vi "main.vi"(0 "Operations":string(tree), 1 "Add":bool, 3 "Delete":bool, 11 "Error In":errorcluster, 12 "Save Data":bool, 13 "Load Data":bool, 14 "Operation List":string(combo)="Add") -> (15 "Error Out":errorcluster)   [LabVIEW 2020, in "Calculator_Using_Objects.lvlib"]
doc: "This VI is to perform the math operations. Whereas the history of the operations will be saved in objects. \nThey can be retrived from the memory during the start of the VI."
uses:
  Calculator_Using_Objects.lvlib
  Typedef's/Q_Operations.ctl
  Typedef's/Data_Cluster.ctl
  Classes/Arithmetic_Operations/Arithmetic_Operations.lvclass
  Typedef's/UserEvent_Operations.ctl
  Classes/Children/Add/Add.lvclass
  Classes/Children/Divide/Divide.lvclass
  Classes/Children/Multiplication/Multiplication.lvclass
  Classes/Children/Subtract/Subtract.lvclass
  Typedef's/Event_Data.ctl
  Typedef's/Object_And_Name_Cluster.ctl
  <vilib>/Utility/error.llb/DialogType.ctl
  <vilib>/Utility/xml.llb/Write to XML File(string).vi
  <vilib>/Utility/xml.llb/Read From XML File(string).vi
panel:
  # "Description:\n1. The classes that were present in the children folder in classes will be automatically loaded into the Operation List box. \n2. Double click any one of it and press add button to add once instance of that particular operation into the Operations box. \n3. Once the operation is clicked the particular instance operation method will be loaded into the subpanel. Where it will have the controls to perform \nthe operations.\n4. The delete button will delete that particular instance of operation in the Operations. \n5. The Save Data button will save all the data instances into a file which can be loaded later. \n6. The Load button will load the data that is already stored in the disc. Loading data will clear all the existing data."
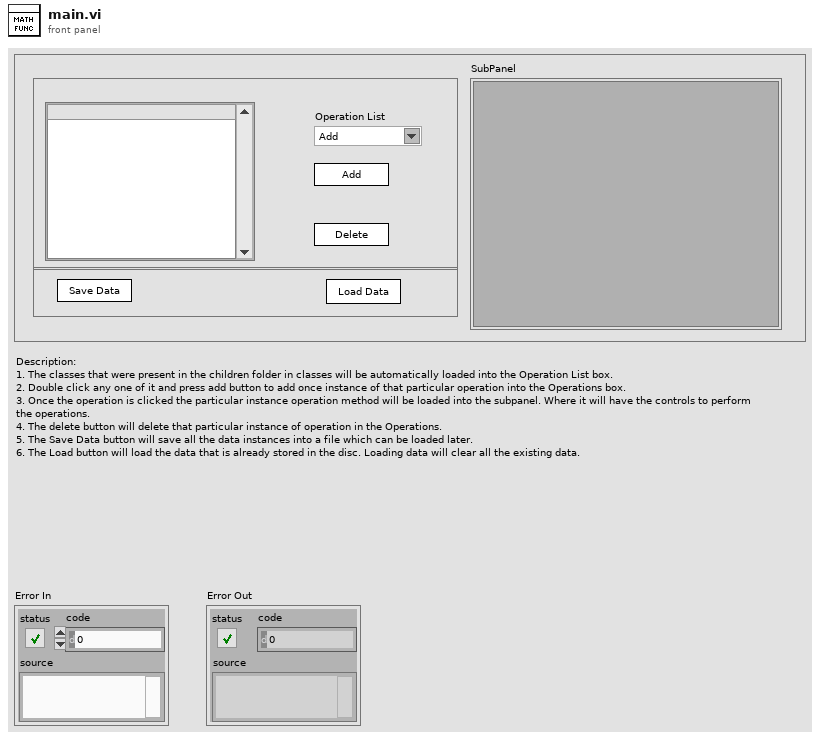
[diagram p1: front panel]
types:
  T1 = typedef "Calculator_Using_Objects.lvlib/UserEvent_Operations.ctl" = enum16{"Create", "Generate", "Get Ref", "Destroy"}
  T2 = typedef "Calculator_Using_Objects.lvlib/Data_Cluster.ctl" = cluster{"Operation Selected":string, "Objects Array":refnum<class "Arithmetic_Operations.lvclass">[], "Prev Row Number":i32, "Num 1":dbl, "Num 2":dbl, "Application Path":path, "Row Number":i32, "Subpanel FP?":bool}
  T3 = typedef "Calculator_Using_Objects.lvlib/Q_Operations.ctl" = enum16{"Create Q", "Enqueue", "Dequeue", "Enqueue N ele", "Enstack N ele", "Flush Q", "Destroy Q"}
  T4 = typedef "Calculator_Using_Objects.lvlib/Event_Data.ctl" = cluster{"Stop Data":bool}
  T5 = typedef "Calculator_Using_Objects.lvlib/Object_And_Name_Cluster.ctl" = cluster{"Tree Entry":string[], "Object Array":refnum<class "Arithmetic_Operations.lvclass">[]}
  T6 = enum16{"open", "replace", "create", "open or create", "replace or create", "replace or create with confirmation"}
  T7 = typedef "DialogType.ctl" = u16
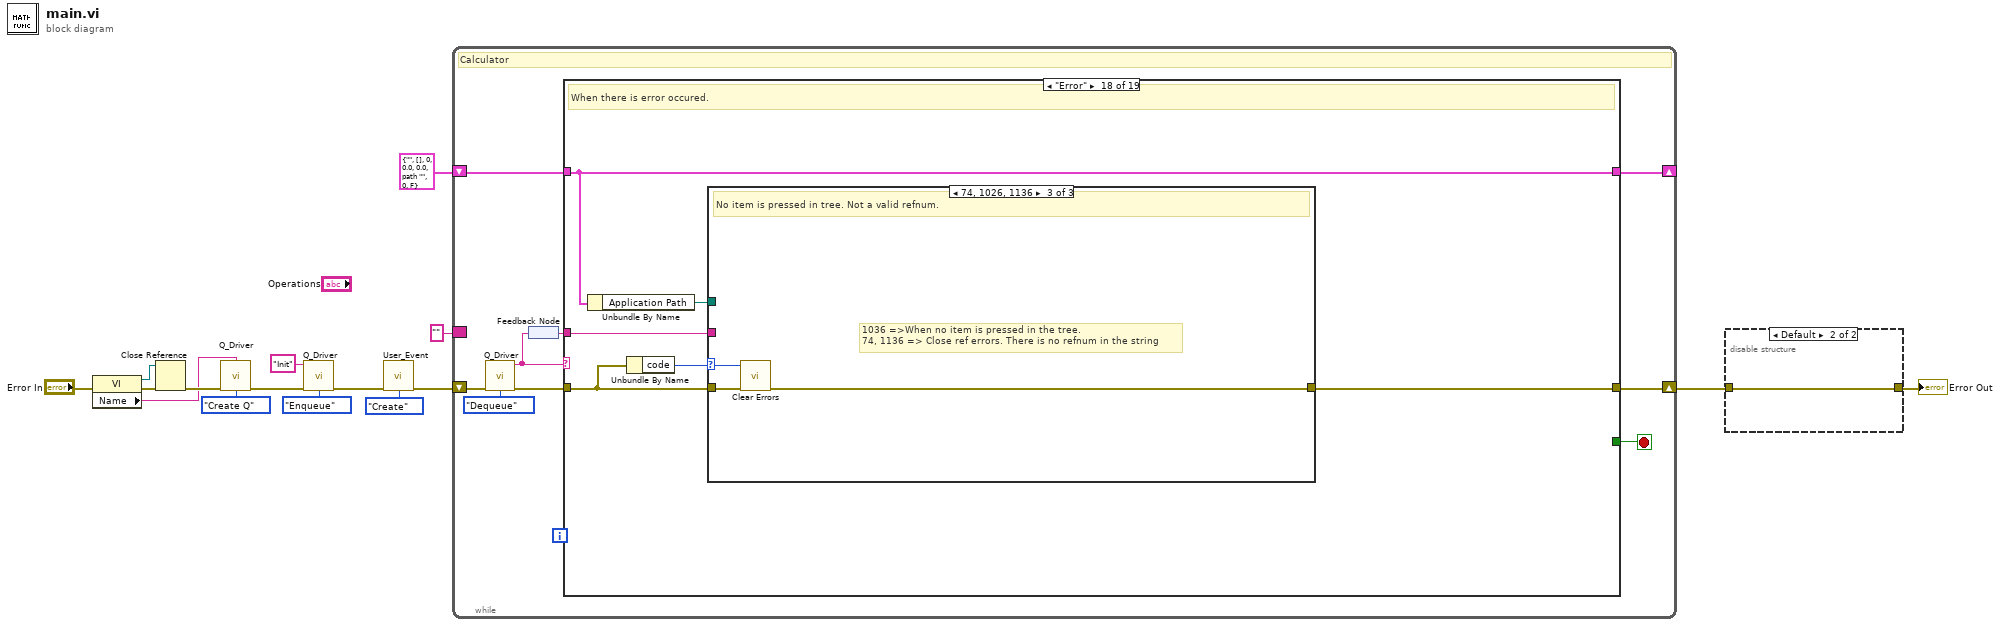
[diagram p0: block diagram]
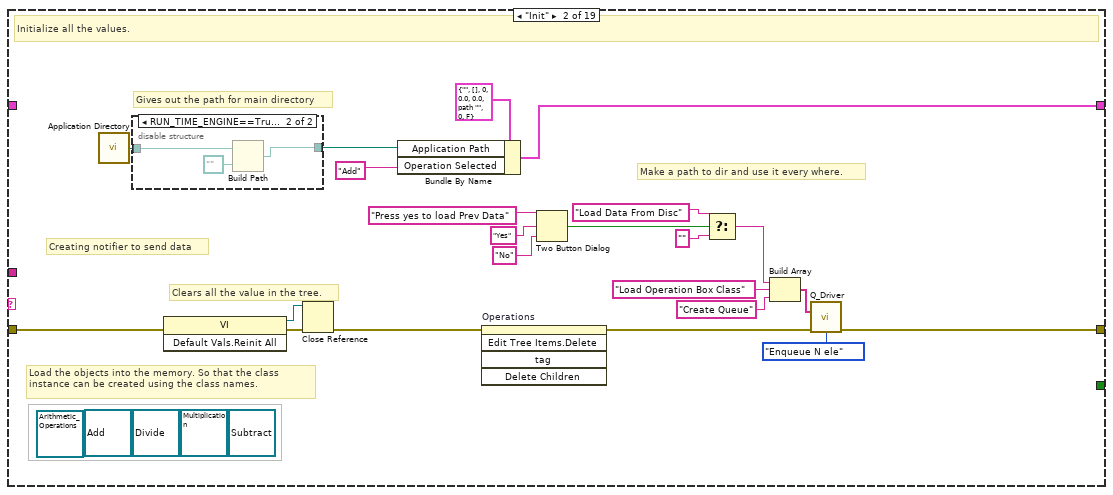
[diagram p3: hidden frame]
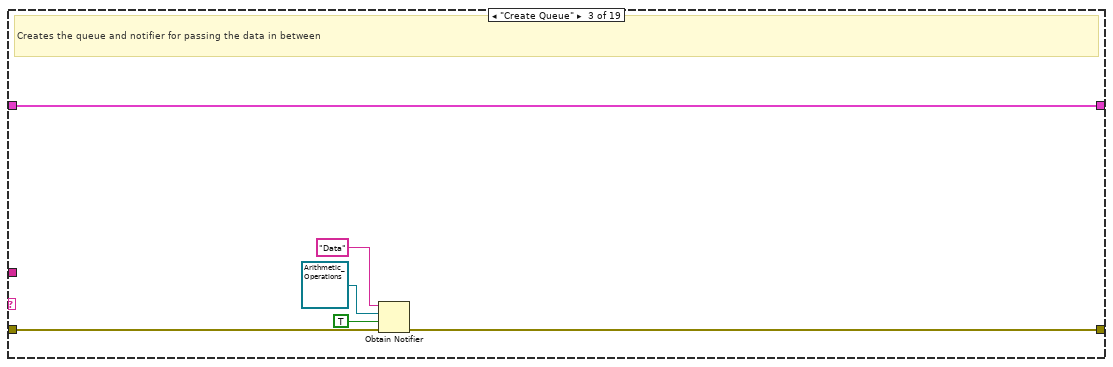
[diagram p5: hidden frame]
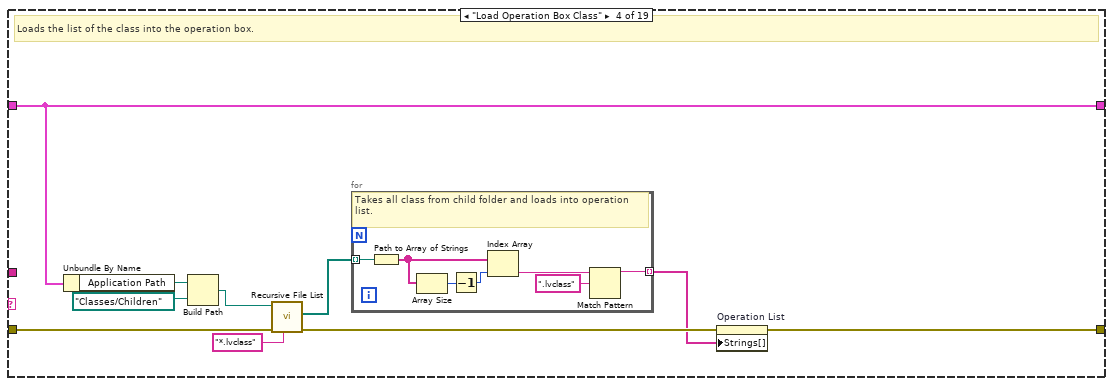
[diagram p6: hidden frame]
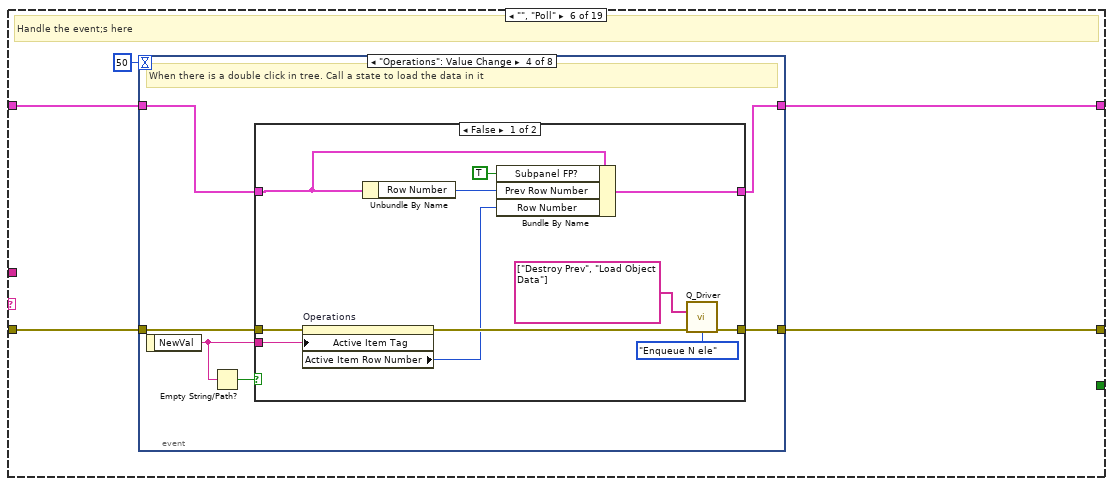
[diagram p8: hidden frame]
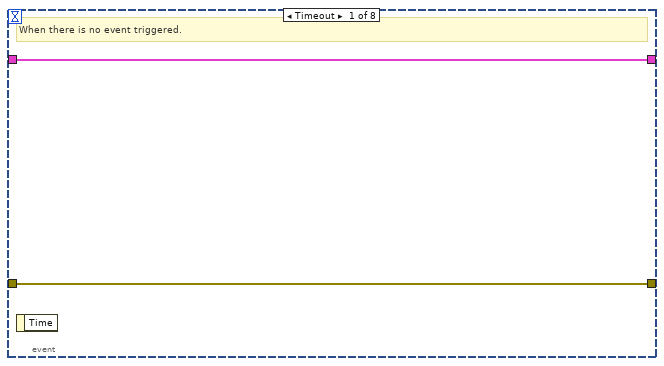
[diagram p9: hidden frame]
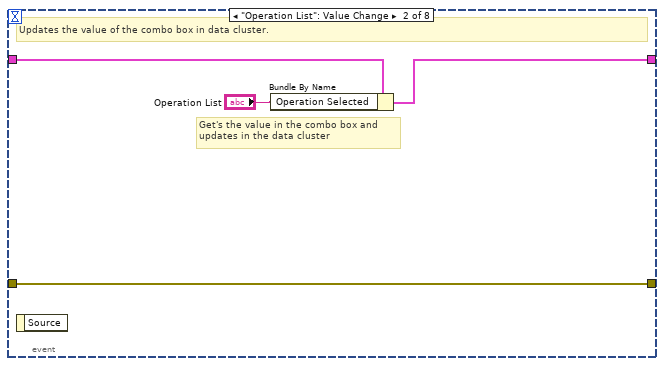
[diagram p10: hidden frame]
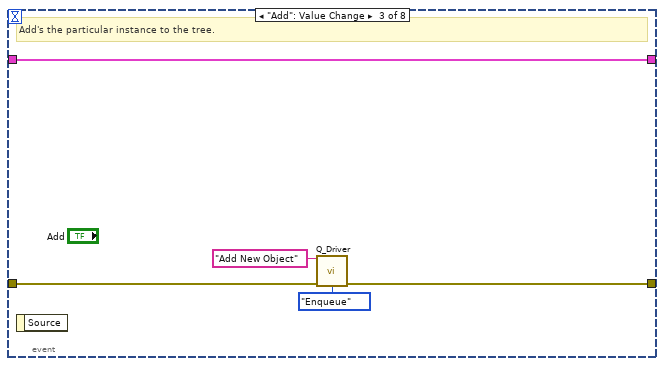
[diagram p11: hidden frame]
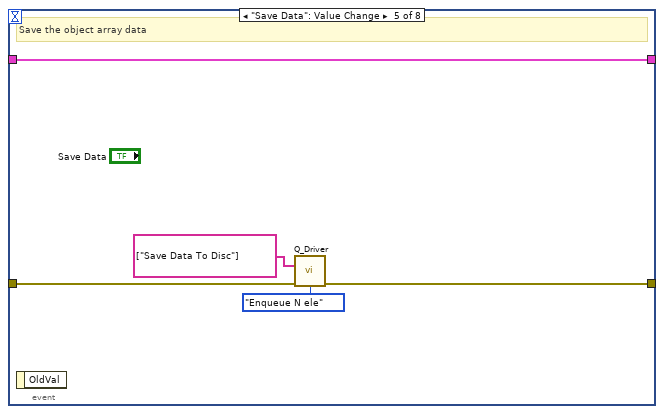
[diagram p13: hidden frame]
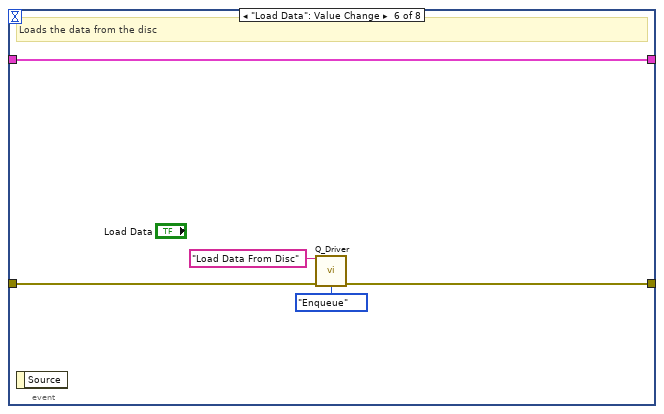
[diagram p14: hidden frame]
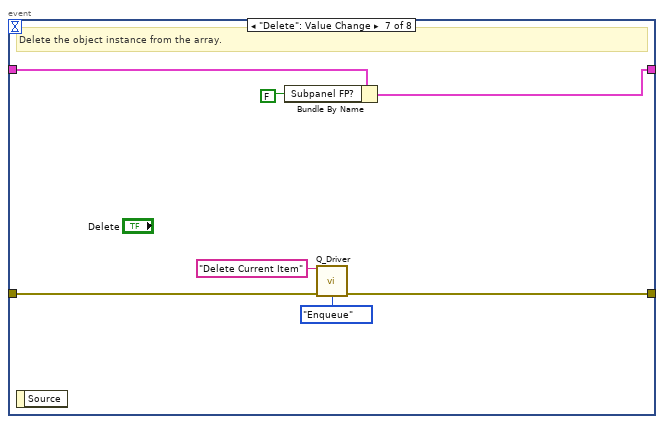
[diagram p15: hidden frame]
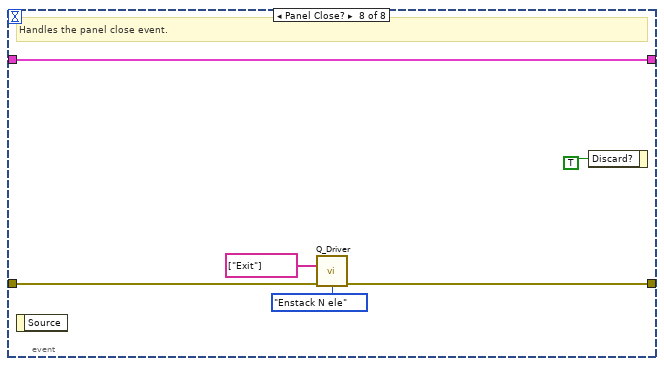
[diagram p16: hidden frame]
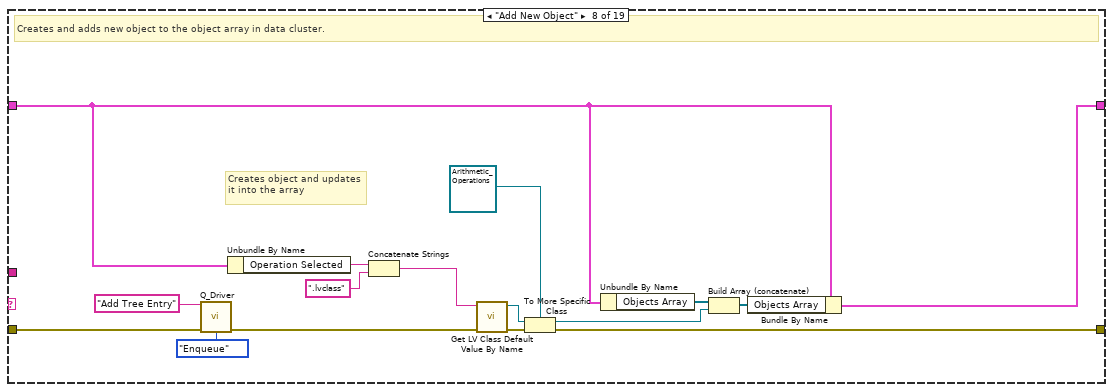
[diagram p18: hidden frame]
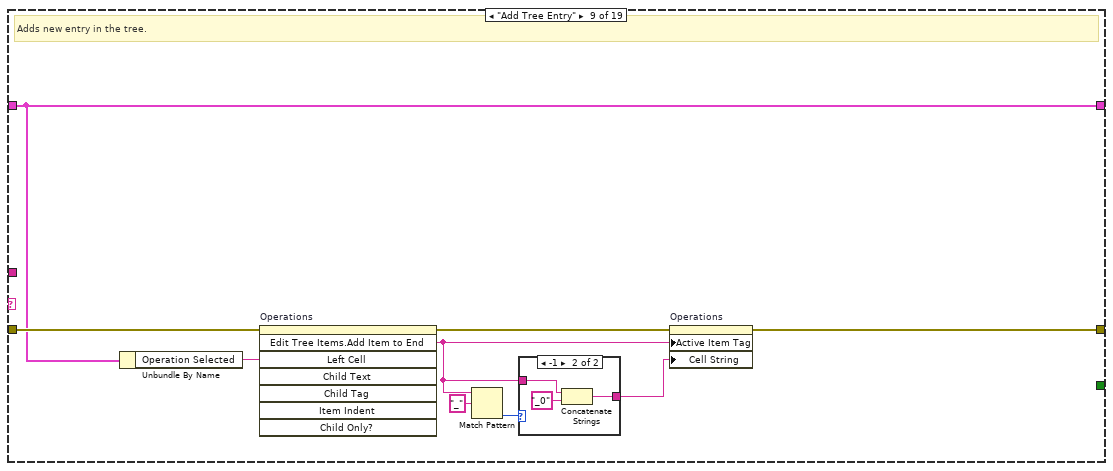
[diagram p19: hidden frame]
diagram:
  n1 = property class="VI"(error in="Error In") -> (reference out=w13:refnum<vi>, error out=w15:errorcluster, "Name"=w10:string)  [unwired: 1 in]
  n2 = Close Reference(reference=w13, error in (no error)=w15) -> (error out=w14:errorcluster)
  n3 = call "Q_Driver.vi"("Name"=w10, "Error In"=w14, "Operations"=Q_Operations."Create Q") -> ("Error Out"=w12:errorcluster)  [unwired: 11 in, 1 out]
  n4 = call "Q_Driver.vi"("State"="Init", "Error In"=w12, "Operations"=Q_Operations."Enqueue") -> ("Error Out"=w9:errorcluster)  [unwired: 11 in, 1 out]
  n5 = call "User_Event.vi"("Error In"=w9, "Enum"=UserEvent_Operations."Create") -> ("Error Out"=w6:errorcluster)  [unwired: 12 in, 1 out]
  n6 = while {
    shift-right: [w22] -> w4
    shift-left: w6 -> [w24]
    shift-right: [w19] -> _
    shift-left: T2 {"Operation Selected"="", "Objects Array"=[], "Prev Row Number"=0, "Num 1"=0.0, "Num 2"=0.0, "Application Path"=path "", "Row Number"=0, "Subpanel FP?"=FALSE} ("Data Cluster") -> [w20]
    border: "" ("Dequeued Element") -> [_]
    stop <- w21 stop-if-true
    # "Calculator"
    n7 = call "Q_Driver.vi"("Error In"=w24, "Operations"=Q_Operations."Dequeue") -> ("Dequeued Element"=w18:string, "Error Out"=w25:errorcluster)  [unwired: 12 in]
    n8 = feedback-in #1(w18) -> ()
    n9 = feedback #1() -> (w17:string)
    n10 = case shown="\"Error\"" w18 {
      tunnel: w25 -> [w27 w37 w54 w69 w78 w82 w138 w154 w163 w172 w198 w201 w211 w251 w259 w267 w281 w286 w330]
      tunnel: [w27 w42 w55 w65 w78 w81 w138 w153 w157 w171 w196 w206 w212 w244 w259 w264 w281 w287 w330] -> w22
      tunnel: [_ _ _ _ _ _ _ _ _ _ _ _ _ _ _ TRUE _ _ _] -> w21
      tunnel: w20 -> [w26 _ w59 w63 w77 w80 w137 w151 w161 w168 w197 w207 w209 w249 w258 w261 w280 w284 w329]
      tunnel: [w26 w33 w59 w63 w77 w79 w137 w148 w161 w169 w195 w207 w210 w245 w258 w261 w280 w284 w329] -> w19
      tunnel: w17 -> [_ _ _ _ _ _ _ _ _ _ _ _ _ _ _ _ _ w282 _]
      frame "/**** Initialize ****/" {
      }
      frame "Init" {
        (unwired) refnum<class "Subtract.lvclass"> refnum ("Subtract.lvclass")
        (unwired) refnum<class "Multiplication.lvclass"> refnum ("Multiplication.lvclass")
        (unwired) refnum<class "Divide.lvclass"> refnum ("Divide.lvclass")
        (unwired) refnum<class "Add.lvclass"> refnum ("Add.lvclass")
        (unwired) refnum<class "Arithmetic_Operations.lvclass"> refnum ("Arithmetic_Operations.lvclass")
        # "Creating notifier to send data"
        # "Load the objects into the memory. So that the class instance can be created using the class names."
        # "Gives out the path for main directory"
        # "Make a path to dir and use it every where."
        # "Clears all the value in the tree."
        # "Initialize all the values."
        n11 = call <vilib>:"Application Directory.vi"() -> ("Application Directory"=w31:path)
        n12 = disable-structure shown="RUN_TIME_ENGINE==True" {
          disable-tunnel: [w50 w51] -> w32
          disable-tunnel: w31 -> [w50 w53]
          frame condition #0 (active) {
          }
          frame condition #1 {
            n13 = Build Path(base path=w53, name or relative path=path "..") -> (appended path=w51:path)
          }
        }
        n14 = invoke class="VI" method="Default Vals.Reinit All"(error in=w37) -> (reference out=w48:refnum<vi>, error out=w49:errorcluster)  [unwired: 2 in, 1 out]
        n15 = Close Reference(reference=w48, error in (no error)=w49) -> (error out=w47:errorcluster)
        n16 = Bundle By Name(cluster=T2 {"Operation Selected"="", "Objects Array"=[], "Prev Row Number"=0, "Num 1"=0.0, "Num 2"=0.0, "Application Path"=path "", "Row Number"=0, "Subpanel FP?"=FALSE} ("Data Cluster"), "Application Path"=w32, "Operation Selected"="Add") -> (w33:T2)
        n17 = invoke on="Operations" class="Tree (strict)" method="Edit Tree Items.Delete"(error in=w47) -> (error out=w43:errorcluster)  [unwired: 4 in, 4 out]
        n18 = Two Button Dialog(message="Press yes to load Prev Data", 1:"No" ("F button name (\"Cancel\")"), 2:"Yes" ("T button name (\"OK\")")) -> (T button?=w41:bool)
        n19 = Select(t="Load Data From Disc", s=w41, f="") -> (s? t:f=w36:string)
        n20 = Build Array(w36, "Load Operation Box Class", "Create Queue") -> (w34:string[])
        n21 = call "Q_Driver.vi"("States[]"=w34, "Error In"=w43, "Operations"=Q_Operations."Enqueue N ele") -> ("Error Out"=w42:errorcluster)  [unwired: 11 in, 1 out]
      }
      frame "Create Queue" {
        # "Creates the queue and notifier for passing the data in between"
        n22 = Obtain Notifier(name (unnamed)="Data", notification data type=refnum<class "Arithmetic_Operations.lvclass"> refnum ("Arithmetic_Operations.lvclass"), create if not found? (T)=TRUE, error in (no error)=w54) -> (error out=w55:errorcluster)  [unwired: 2 out]
      }
      frame "Load Operation Box Class" {
        # "Loads the list of the class into the operation box."
        n23 = Unbundle By Name(w63) -> ("Application Path"=w61:path)
        n24 = Build Path(base path=w61, name or relative path=path "Classes/Children") -> (appended path=w60:path)
        n25 = call <vilib>:"Recursive File List.vi"("pattern"="*.lvclass", "error in (no error)"=w69, "Folder Path"=w60) -> ("error out"=w68:errorcluster, "All Files in Dir"=w66:path[])  [unwired: 4 in, 3 out]
        n26 = for {
          tunnel: w66 -> [w76] mode=indexing
          tunnel: [w70] -> w64 mode=indexing
          # "Takes all class from child folder and loads into operation list."
          n27 = Path to Array of Strings(0:w76) -> (2:w74:string[])  [unwired: 1 out]
          n28 = Array Size(array=w74) -> (size(s)=w75:i32)
          n29 = Decrement(x=w75) -> (x-1=w73:i32)
          n30 = Index Array(array=w74, index=w73) -> (element=w72:string)
          n31 = Match Pattern(string=w72, regular expression=".lvclass") -> (before substring=w70:string)  [unwired: 1 in, 3 out]
        }
        n32 = property on="Operation List" class="CmbBox"(error in=w68, "Strings[]"=w64) -> (error out=w65:errorcluster)  [unwired: 1 in, 1 out]
      }
      frame "/****Events*****/" {
      }
      frame "", "Poll" {
        # "Handle the event;s here"
        n33 = event shown="[3] \"Operations\": Value Change" {
          selector: _ -> [_ _ _ _ _ _ _ _]
          dyn-events: _ -> [_ _ _ _ _ _ _ _]
          timeout: 50 -> [_ _ _ _ _ _ _ _]
          tunnel: w82 -> [w85 w89 w94 w99 w118 w123 w130 w136]
          tunnel: [w85 w89 w92 w100 w116 w121 w128 w134] -> w81
          tunnel: [w84 w87 w93 w96 w117 w122 w125 w131] -> w79
          tunnel: w80 -> [w84 w88 w93 w97 w117 w122 w129 w131]
          event Timeout {
            # "When there is no event triggered."
            n34 = event-data() -> ()  [unwired: 1 in, 1 out]
          }
          event "Operation List": Value Change {
            # "Get's the value in the combo box and\nupdates in the data cluster"
            # "Updates the value of the combo box in data cluster."
            n35 = event-data() -> ()  [unwired: 1 in, 1 out]
            n36 = Bundle By Name(cluster=w88, "Operation Selected"="Operation List") -> (w87:T2)
          }
          event "Add": Value Change {
            # "Add's the particular instance to the tree."
            n37 = event-data() -> ()  [unwired: 1 in, 1 out]
            n38 = call "Q_Driver.vi"("State"="Add New Object", "Error In"=w94, "Operations"=Q_Operations."Enqueue") -> ("Error Out"=w92:errorcluster)  [unwired: 11 in, 1 out]
          }
          event "Operations": Value Change {
            # "When there is a double click in tree. Call a state to load the data in it"
            n39 = event-data() -> ("NewVal"=w98:string)  [unwired: 1 in]
            n40 = Empty String/Path?(string/path=w98) -> (empty?=w95:bool)
            n41 = case shown="False" w95 {
              tunnel: [w111 w113] -> w100
              tunnel: [w110 w112] -> w96
              tunnel: w99 -> [w106 w113]
              tunnel: w98 -> [w104 _]
              tunnel: w97 -> [w101 w112]
              frame False {
                n42 = property on="Operations" class="Tree (strict)"(error in=w106, "Active Item Tag"=w104) -> (error out=w109:errorcluster, "Active Item Row Number"=w108:i32)  [unwired: 1 in, 1 out]
                n43 = Unbundle By Name(w101) -> ("Row Number"=w107:i32)
                n44 = Bundle By Name(cluster=w101, "Subpanel FP?"=TRUE, "Prev Row Number"=w107, "Row Number"=w108) -> (w110:T2)
                n45 = call "Q_Driver.vi"("States[]"=string[] ["Destroy Prev", "Load Object Data"], "Error In"=w109, "Operations"=Q_Operations."Enqueue N ele") -> ("Error Out"=w111:errorcluster)  [unwired: 11 in, 1 out]
              }
              frame True {
              }
            }
          }
          event "Save Data": Value Change {
            # "Save the object array data"
            n46 = event-data() -> ()  [unwired: 1 in, 1 out]
            n47 = call "Q_Driver.vi"("States[]"=string[] ["Save Data To Disc"], "Error In"=w118, "Operations"=Q_Operations."Enqueue N ele") -> ("Error Out"=w116:errorcluster)  [unwired: 11 in, 1 out]
          }
          event "Load Data": Value Change {
            # "Loads the data from the disc"
            n48 = event-data() -> ()  [unwired: 1 in, 1 out]
            n49 = call "Q_Driver.vi"("State"="Load Data From Disc", "Error In"=w123, "Operations"=Q_Operations."Enqueue") -> ("Error Out"=w121:errorcluster)  [unwired: 11 in, 1 out]
          }
          event "Delete": Value Change {
            # "Delete the object instance from the array."
            n50 = event-data() -> ()  [unwired: 1 in, 1 out]
            n51 = Bundle By Name(cluster=w129, "Subpanel FP?"=FALSE) -> (w125:T2)
            n52 = call "Q_Driver.vi"("State"="Delete Current Item", "Error In"=w130, "Operations"=Q_Operations."Enqueue") -> ("Error Out"=w128:errorcluster)  [unwired: 11 in, 1 out]
          }
          event Panel Close? {
            # "Handles the panel close event."
            n53 = event-data() -> ()  [unwired: 1 in, 1 out]
            n54 = call "Q_Driver.vi"("States[]"=string[] ["Exit"], "Error In"=w136, "Operations"=Q_Operations."Enstack N ele") -> ("Error Out"=w134:errorcluster)  [unwired: 11 in, 1 out]
            n55 = event-data("Discard?"=TRUE) -> ()  [unwired: 1 in, 1 out]
          }
        }
      }
      frame "/**** Functionalities ***/" {
      }
      frame "Add New Object" {
        # "Creates object and updates it into the array"
        # "Creates and adds new object to the object array in data cluster."
        n56 = call "Q_Driver.vi"("State"="Add Tree Entry", "Error In"=w154, "Operations"=Q_Operations."Enqueue") -> ("Error Out"=w146:errorcluster)  [unwired: 11 in, 1 out]
        n57 = Unbundle By Name(w151) -> ("Operation Selected"=w141:string)
        n58 = Concatenate Strings(w141, ".lvclass") -> (w139:string)
        n59 = call <vilib>:"Get LV Class Default Value By Name.vi"("error in (no error)"=w146, "class name"=w139) -> ("error out"=w143:errorcluster, "object"=w142:refnum<class>)  [unwired: 8 in]
        n60 = To More Specific Class(target class=refnum<class "Arithmetic_Operations.lvclass"> refnum ("Arithmetic_Operations.lvclass"), reference=w142, error in=w143) -> (specific class reference=w149:refnum<class "Arithmetic_Operations.lvclass">, error out=w153:errorcluster)
        n61 = Unbundle By Name(w151) -> ("Objects Array"=w150:refnum<class "Arithmetic_Operations.lvclass">[])
        n62 = Build Array (concatenate)(w150, w149) -> (w147:refnum<class "Arithmetic_Operations.lvclass">[])
        n63 = Bundle By Name(cluster=w151, "Objects Array"=w147) -> (w148:T2)
      }
      frame "Add Tree Entry" {
        # "Adds new entry in the tree."
        n64 = Unbundle By Name(w161) -> ("Operation Selected"=w162:string)
        n65 = invoke on="Operations" class="Tree (strict)" method="Edit Tree Items.Add Item to End"(error in=w163, "Left Cell"=w162) -> (error out=w158:errorcluster, "Edit Tree Items:Add Item to End"=w156:string)  [unwired: 6 in, 6 out]
        n66 = Match Pattern(string=w156, regular expression="_") -> (offset past match=w159:i32)  [unwired: 1 in, 3 out]
        n67 = case shown="-1" w159 {
          tunnel: w156 -> [w164 w166]
          tunnel: [w164 w165] -> w155
          frame 0, Default {
          }
          frame -1 {
            n68 = Concatenate Strings(w166, "_0" ("string")) -> (w165:string)
          }
        }
        n69 = property on="Operations" class="Tree (strict)"(error in=w158, "Active Item Tag"=w156, "Cell String"=w155) -> (error out=w157:errorcluster)  [unwired: 1 in, 1 out]
      }
      frame "Destroy Prev" {
        # "Destroy's the prev operation using the event."
        n70 = First Call?() -> (First Call?: T/F=w170:bool)
        n71 = case shown="False" w170 {
          tunnel: w172 -> [w185 w187]
          tunnel: [w173 w187] -> w171
          tunnel: w168 -> [w181 w186]
          tunnel: [w175 w186] -> w169
          frame False {
            # "After first call do these operation."
            n72 = invoke on="SubPanel" class="SubPnl" method="Remove VI"(error in=w185) -> (error out=w184:errorcluster)  [unwired: 2 in, 2 out]
            n73 = Unbundle By Name(w181) -> ("Objects Array"=w178:refnum<class "Arithmetic_Operations.lvclass">[], "Prev Row Number"=w176:i32)
            n74 = call "User_Event.vi"("Event Data"=T4 {"Stop Data"=TRUE}, "Error In"=w184, "Enum"=UserEvent_Operations."Generate") -> ("Error Out"=w179:errorcluster)  [unwired: 11 in, 1 out]
            n75 = Index Array(array=w178, index=w176) -> (element=w180:refnum<class "Arithmetic_Operations.lvclass">)
            n76 = call-dynamic "Get_Data.vi"("Arithmetic_Operations in"=w180, "Error In"=w179) -> ("Arithmetic_Operations out"=w177:refnum<class "Arithmetic_Operations.lvclass">, "Error Out"=w173:errorcluster)  [unwired: 12 in]
            n77 = Replace Array Subset(array=w178, new element=w177, index=w176) -> (w174:refnum<class "Arithmetic_Operations.lvclass">[])
            n78 = Bundle By Name(cluster=w181, "Objects Array"=w174) -> (w175:T2)
          }
          frame True {
            # "During first call do nothing."
          }
        }
      }
      frame "Load Object Data" {
        # "Loads the object data into the front panel."
        n79 = property on="Operations" class="Tree (strict)"(error in=w198) -> (error out=w188:errorcluster, "Active Item Row Number"=w193:i32)  [unwired: 1 in, 1 out]
        n80 = Unbundle By Name(w197) -> ("Objects Array"=w194:refnum<class "Arithmetic_Operations.lvclass">[])
        n81 = Index Array(array=w194, index=w193) -> (element=w190:refnum<class "Arithmetic_Operations.lvclass">)
        n82 = control-ref of="SubPanel"() -> (w189:refnum<vi>)
        n83 = call-dynamic "Talker.vi"("Arithmetic_Operations in"=w190, "Subpanel Ref"=w189, "Error In"=w188) -> ("Arithmetic_Operations out"=w191:refnum<class "Arithmetic_Operations.lvclass">, "Error Out"=w196:errorcluster)  [unwired: 11 in]
        n84 = Replace Array Subset(array=w194, new element=w191, index=w193) -> (w192:refnum<class "Arithmetic_Operations.lvclass">[])
        n85 = Bundle By Name(cluster=w197, "Objects Array"=w192) -> (w195:T2)
      }
      frame "Save Data To Disc" {
        # "Save's the object array data into the file system."
        n86 = property on="Operations" class="Tree (strict)"(error in=w201) -> (error out=w202:errorcluster, "All Tags"=w200:string[])  [unwired: 1 in, 1 out]
        n87 = Unbundle By Name(w207) -> ("Objects Array"=w199:refnum<class "Arithmetic_Operations.lvclass">[])
        n88 = Bundle By Name(cluster=T5 {"Tree Entry"=[], "Object Array"=[]} ("Object and Name Array"), "Object Array"=w199, "Tree Entry"=w200) -> (w203:T5)
        n89 = Flatten To XML(6:w203) -> (2:w205:string)
        n90 = call-poly <vilib>:"Write to XML File.vi"("error in (no error)"=w202, "XML Input"=w205) -> ("error out"=w206:errorcluster)  [unwired: 7 in, 2 out]
      }
      frame "Load Data From Disc" {
        # "Loads the data that is stored in the disc storage"
        n91 = invoke on="Operations" class="Tree (strict)" method="Edit Tree Items.Delete"(error in=w211) -> (error out=w208:errorcluster)  [unwired: 4 in, 4 out]
        n92 = call-poly <vilib>:"Read From XML File.vi"("error in (no error)"=w208) -> ("error out"=w219:errorcluster, "XML Elements"=w217:string)  [unwired: 8 in, 1 out]
        n93 = Unflatten From XML(xml string=w217, type=T5 {"Tree Entry"=[], "Object Array"=[]} ("Object and Name Array"), error in (no error)=w219) -> (value=w216:T5, error out=w218:errorcluster)
        n94 = Unbundle By Name(w216) -> ("Object Array"=w215:refnum<class "Arithmetic_Operations.lvclass">[], "Tree Entry"=w214:string[])
        n95 = Bundle By Name(cluster=w209, "Objects Array"=w215) -> (w210:T2)
        n96 = for {
          shift-right: [w232] -> w212
          shift-left: w218 -> [w233]
          tunnel: w214 -> [w229] mode=indexing
          # "Add all elements to tree"
          n97 = Match Pattern(string=w229, regular expression="_") -> (offset past match=w231:i32)  [unwired: 1 in, 3 out]
          n98 = Match Pattern(string=w229, regular expression="_0") -> (before substring=w221:string, offset past match=w227:i32)  [unwired: 1 in, 2 out]
          n99 = case shown="-1" w231 {
            tunnel: w229 -> [w238 w240]
            tunnel: [w238 w239] -> w220
            frame 0, Default {
            }
            frame -1 {
              n100 = Concatenate Strings(w240, "_0" ("string")) -> (w239:string)
            }
          }
          n101 = Less Than 0?(x=w227) -> (x < 0?=w226:bool)
          n102 = Select(t=w221, s=w226, f=w220) -> (s? t:f=w223:string)
          n103 = Match Pattern(string=w223, regular expression="_") -> (offset past match=w224:i32)  [unwired: 1 in, 3 out]
          n104 = case shown="-1" w224 {
            tunnel: w223 -> [w234 w236]
            tunnel: [w234 w235] -> w222
            frame 0, Default {
            }
            frame -1 {
              n105 = Concatenate Strings(w236, "_0" ("string")) -> (w235:string)
            }
          }
          n106 = invoke on="Operations" class="Tree (strict)" method="Edit Tree Items.Add Item to End"(error in=w233, "Left Cell"=w222, "Child Tag"=w223) -> (error out=w232:errorcluster)  [unwired: 5 in, 7 out]
        }
      }
      frame "Delete Current Item" {
        # "Deletes the current selected item from the table"
        n107 = property on="Operations" class="Tree (strict)"(error in=w251) -> (error out=w250:errorcluster, "Active Item Tag"=w243:string, "Active Item Row Number"=w247:i32)  [unwired: 1 in, 1 out]
        n108 = Unbundle By Name(w249) -> ("Objects Array"=w248:refnum<class "Arithmetic_Operations.lvclass">[])
        n109 = Delete From Array(array=w248, index=w247) -> (array with subset deleted=w246:refnum<class "Arithmetic_Operations.lvclass">[])  [unwired: 1 in, 1 out]
        n110 = Empty String/Path?(string/path=w243) -> (empty?=w242:bool)
        n111 = Bundle By Name(cluster=w249, "Objects Array"=w246) -> (w245:T2)
        n112 = case shown="True" w242 {
          tunnel: w250 -> [w255 w257]
          tunnel: [w252 w257] -> w244
          tunnel: w243 -> [w254 _]
          frame False {
            # "Destroy the current \noperation"
            # "When there is value in active tag"
            n113 = invoke on="Operations" class="Tree (strict)" method="Edit Tree Items.Delete"(error in=w255, "tag"=w254) -> (error out=w253:errorcluster)  [unwired: 3 in, 4 out]
            n114 = invoke on="SubPanel" class="SubPnl" method="Remove VI"(error in=w253) -> (error out=w252:errorcluster)  [unwired: 2 in, 2 out]
          }
          frame True {
            # "When there is no value in active tag"
            n115 = One Button Dialog(message="There is no Item selected. \nSelect any one item and press delete") -> ()  [unwired: 1 in, 1 out]
          }
        }
      }
      frame "/***** Exit******/" {
      }
      frame "Exit" {
        # "Generate a user event and stop the \nUI vi that is running"
        # "Destroy all the events and other's in created in program ."
        # "Handles the exit state"
        n116 = Unbundle By Name(w261) -> ("Subpanel FP?"=w260:bool)
        n117 = case "Close running FP in Subpanel" shown="True" w260 {
          tunnel: w267 -> [w269 w279]
          tunnel: [w269 w272] -> w262
          frame False {
          }
          frame True {
            n118 = call "User_Event.vi"("Event Data"=T4 {"Stop Data"=TRUE}, "Error In"=w279, "Enum"=UserEvent_Operations."Generate") -> ("Error Out"=w278:errorcluster)  [unwired: 11 in, 1 out]
            n119 = Obtain Notifier(name (unnamed)="Data", notification data type=refnum<class "Arithmetic_Operations.lvclass"> refnum ("Arithmetic_Operations.lvclass"), error in (no error)=w278) -> (notifier out=w271:refnum<notifier>, error out=w275:errorcluster)  [unwired: 1 in, 1 out]
            n120 = Wait on Notification(notifier=w271, ignore previous (F)=TRUE, error in (no error)=w275) -> (error out=w272:errorcluster)  [unwired: 1 in, 3 out]
          }
        }
        n121 = call "User_Event.vi"("Error In"=w262, "Enum"=UserEvent_Operations."Destroy") -> ("Error Out"=w266:errorcluster)  [unwired: 12 in, 1 out]
        n122 = call "Q_Driver.vi"("Error In"=w266, "Operations"=Q_Operations."Destroy Q") -> ("Error Out"=w264:errorcluster)  [unwired: 12 in, 1 out]
      }
      frame "/**** Error States ****/" {
      }
      frame "Error" {
        # "When there is error occured."
        n123 = Unbundle By Name(w284) -> ("Application Path"=w283:path)
        n124 = Unbundle By Name(w286) -> ("code"=w285:i32)
        n125 = case shown="74, 1026, 1136" w285 {
          selector: w285 -> [w288 w323 w326]
          tunnel: [w289 w322 w327] -> w287
          tunnel: w286 -> [w291 w325 w328]
          tunnel: w283 -> [w290 _ _]
          tunnel: w282 -> [_ _ _]
          frame 0, Default {
            # "Handle error with simple error handler."
            n126 = disable-structure shown="RUN_TIME_ENGINE==True" {
              disable-tunnel: w291 -> [w312 w318]
              disable-tunnel: w290 -> [w311 _]
              disable-tunnel: [w297 w315] -> w289
              disable-tunnel: w288 -> [w292 _]
              frame condition #0 {
                w304 = "\r\n"
                # "When ran with the exe"
                n127 = Unbundle By Name(w312) -> ("source"=w305:string)
                n128 = call <vilib>:"Clear Errors.vi"("error in (no error)"=w312, "specific error code to clear (0: all)"=w292) -> ("error out"=w293:errorcluster)  [unwired: 4 in, 1 out]
                n129 = Build Path(base path=w311, name or relative path=path "Data/ErrorLog.txt") -> (appended path=w308:path)
                n130 = Open/Create/Replace File(file path (use dialog)=w308, error in=w293, operation (0:open)=T6."open or create") -> (refnum out=w306:refnum<file>, error out=w310:errorcluster)  [unwired: 3 in, 1 out]
                n131 = Read from Text File(file (use dialog)=w306, error in=w310) -> (refnum out=w301:refnum<file>, text=w303:string, error out=w307:errorcluster)  [unwired: 2 in, 1 out]
                n132 = Concatenate Strings(w303, w304, w304, w305) -> (w300:string)
                n133 = Write to Text File(file (use dialog)=w301, text=w300, error in=w307) -> (refnum out=w299:refnum<file>, error out=w302:errorcluster)  [unwired: 1 in, 1 out]
                n134 = One Button Dialog(message="Some error has occured. Error details has been saved in a file. \nPress OK to stop the program") -> ()  [unwired: 1 in, 1 out]
                n135 = Close File(refnum=w299, error in=w302) -> (error out=w313:errorcluster)  [unwired: 1 out]
                n136 = call "Q_Driver.vi"("States[]"=string[] ["Exit"], "Error In"=w313, "Operations"=Q_Operations."Enstack N ele") -> ("Error Out"=w297:errorcluster)  [unwired: 11 in, 1 out]
              }
              frame condition #1 (active) {
                w316 = T7 2 items=["no dialog", "OK message", "continue or stop message", "OK message + warnings", "continue/stop + warnings"] ("type of dialog (OK msg:1)")
                # "When ran with developement env"
                n137 = call <vilib>:"Simple Error Handler.vi"("type of dialog (OK msg:1)"=w316, "error in (no error)"=w318) -> ("code out"=w314:i32, "error out"=w317:errorcluster)  [unwired: 3 in, 3 out]
                n138 = call <vilib>:"Clear Errors.vi"("error in (no error)"=w317, "specific error code to clear (0: all)"=w314) -> ("error out"=w315:errorcluster)  [unwired: 4 in, 1 out]
              }
            }
          }
          frame 43 {
            # "Item is can by the user. Selection of file during pop up stopped"
            n139 = call <vilib>:"Clear Errors.vi"("error in (no error)"=w325, "specific error code to clear (0: all)"=w323) -> ("error out"=w324:errorcluster)  [unwired: 4 in, 1 out]
            n140 = One Button Dialog(message="Item selection cancelled. \nPress Ok to stop") -> ()  [unwired: 1 in, 1 out]
            n141 = call "Q_Driver.vi"("States[]"=string[] ["Exit"], "Error In"=w324, "Operations"=Q_Operations."Enstack N ele") -> ("Error Out"=w322:errorcluster)  [unwired: 11 in, 1 out]
          }
          frame 74, 1026, 1136 {
            # "1036 =>When no item is pressed in the tree.\n74, 1136 => Close ref errors. There is no refnum in the string"
            # "No item is pressed in tree. Not a valid refnum."
            n142 = call <vilib>:"Clear Errors.vi"("error in (no error)"=w328, "specific error code to clear (0: all)"=w326) -> ("error out"=w327:errorcluster)  [unwired: 4 in, 1 out]
          }
        }
      }
      frame "Developer Error", Default {
        # "When there is some error made by developer"
      }
    }
  }
  n143 = disable-structure shown="Default" {
    disable-tunnel: w4 -> [w334 w335]
    disable-tunnel: [w332 w335] -> w2
    frame condition #0 {
      n144 = invoke class="VI" method="FP.Close"(error in=w334) -> (reference out=w331:refnum<vi>, error out=w333:errorcluster)  [unwired: 2 in, 1 out]
      n145 = Close Reference(reference=w331, error in (no error)=w333) -> (error out=w332:errorcluster)
    }
    frame condition #1 (active) {
    }
  }
  "Error Out" <- w2
